vi "Manipulate_TDMS_files.vi"() -> ()   [LabVIEW 2015]
panel:
  in  "Group Name":bool
  in  "New Group Name":string
  out "Adding":bool
  out "Deleting":bool
  out "name2":string
  out "name 1":string
  in  "Add Button":bool
  in  "Open Button 2":bool
  in  "Listbox 2":i32[](listbox)=[9] caption="FreeRun_Beam_Tests_Int_Scint_2Apr2018.tdms"
  out "group names 2":string[](array[string])
  out "selected path 2":path caption="selected path"
  in  "Stop Button":bool
  in  "Remove Button":bool
  in  "Listbox":i32[](listbox)=[9] caption="FreeRun_Int_scint_new.tdms"
  in  "Open Button":bool
  out "group names":string[](array[string])
  out "selected path":path
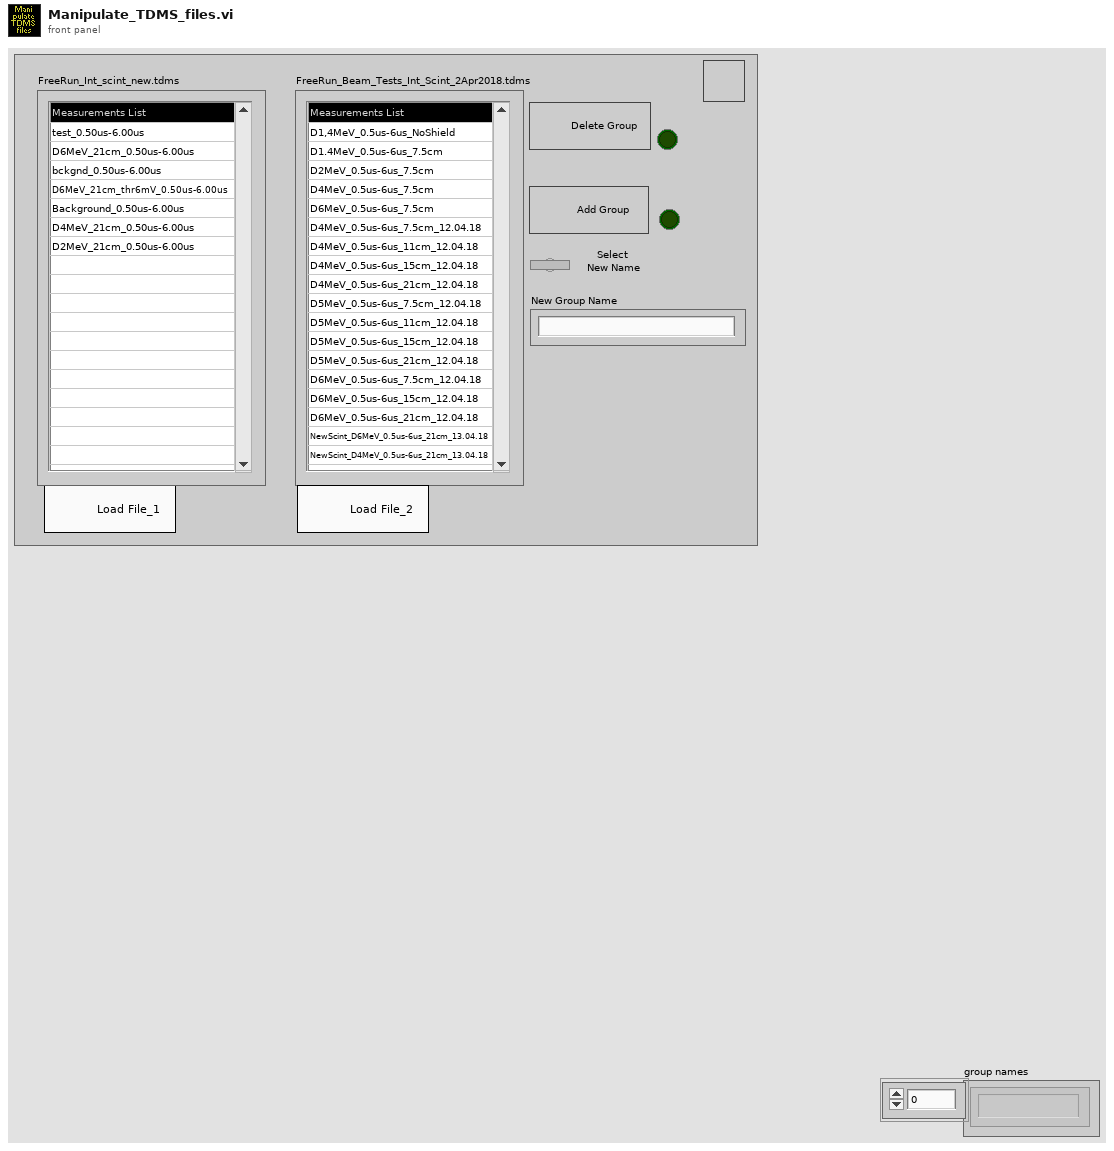
[diagram p1: front panel]
types:
  T1 = enum16{"open", "open or create", "create or replace", "create", "open (read-only)"}
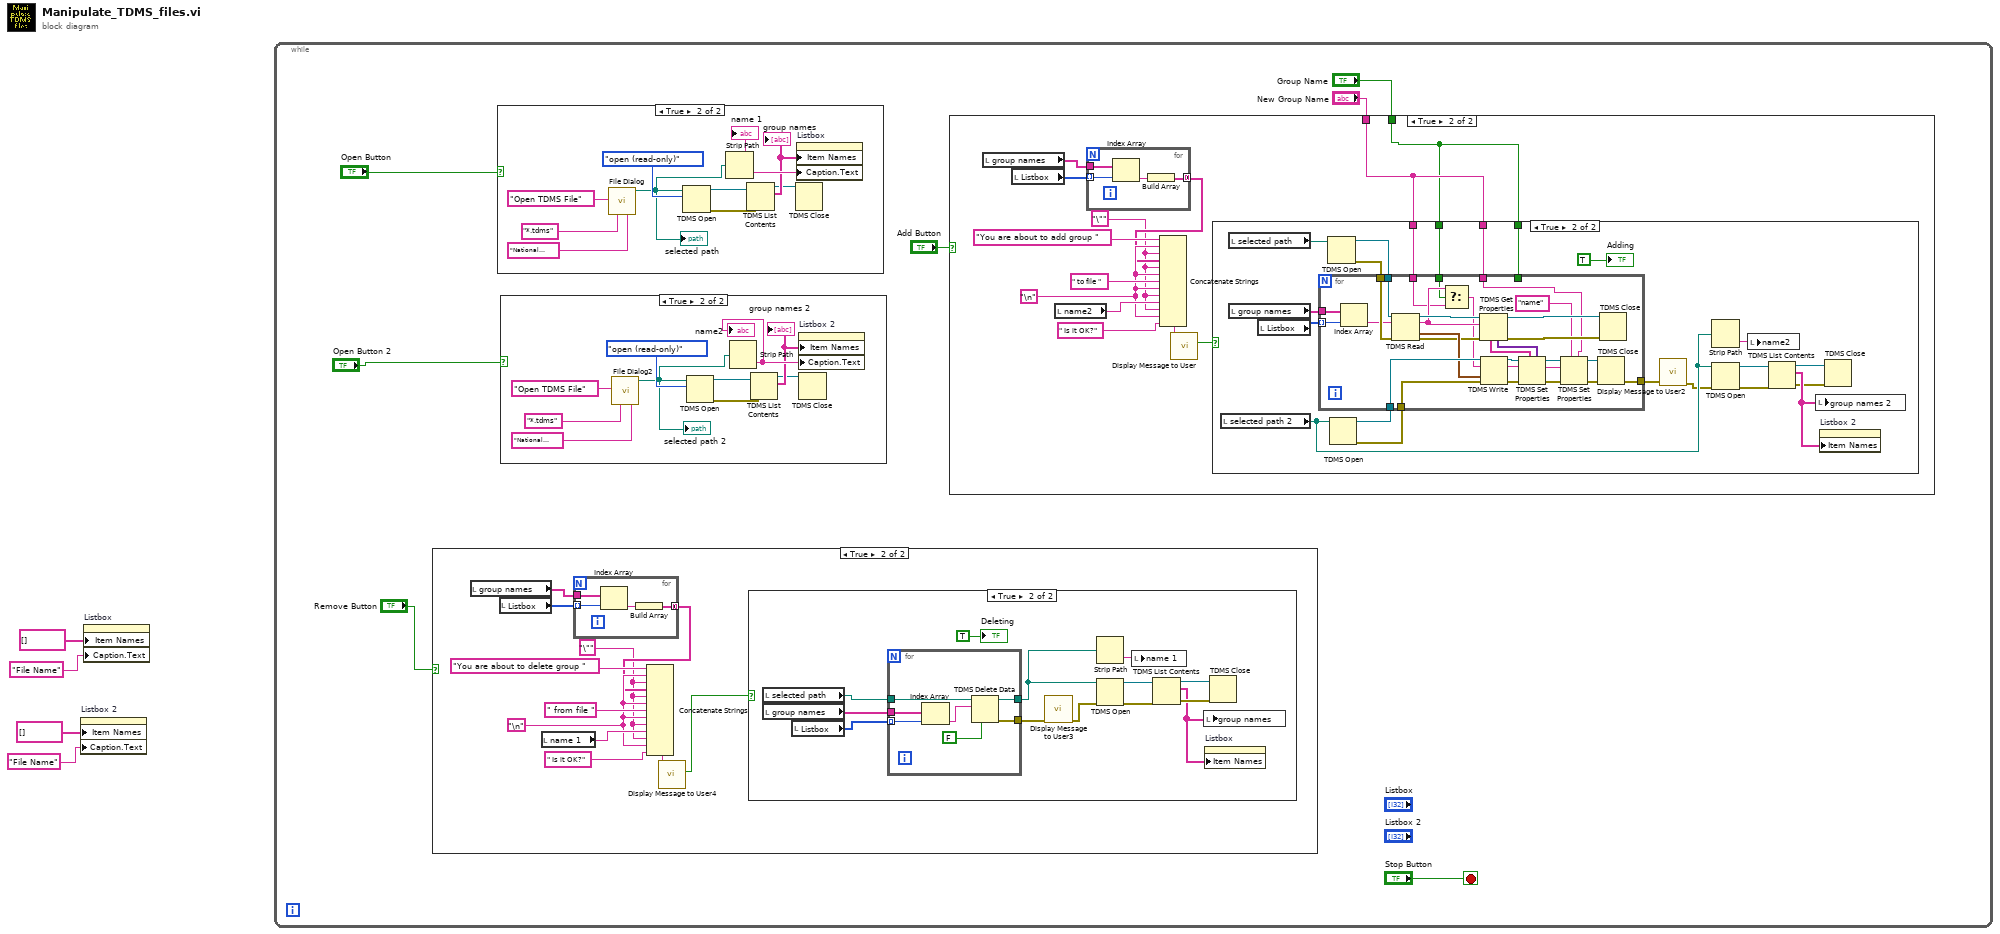
[diagram p0: block diagram]
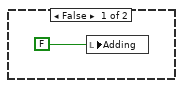
[diagram p2: hidden frame]
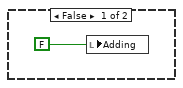
[diagram p3: hidden frame]
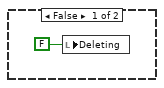
[diagram p5: hidden frame]
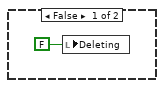
[diagram p6: hidden frame]
diagram:
  n1 = property on="Listbox 2" class="LstBox (strict)"("Item Names"=string[] [], "Caption.Text"="File Name") -> ()  [unwired: 2 in, 2 out]
  n2 = property on="Listbox" class="LstBox (strict)"("Item Names"=string[] [], "Caption.Text"="File Name") -> ()  [unwired: 2 in, 2 out]
  n3 = while {
    stop <- "Stop Button" stop-if-true
    n4 = case shown="True" "Remove Button" {
      frame False {
        n5 = local write "Deleting"(FALSE ("Deleting")) -> ()
      }
      frame True {
        w93 = "\""
        w95 = "\n"
        n6 = local read "group names"() -> (w101:string[])
        n7 = local read "Listbox"() -> (w100:i32[])
        n8 = local read "name 1"() -> (w99:string)
        n9 = for {
          tunnel: w101 -> [w106]
          tunnel: w100 -> [w105] mode=indexing
          tunnel: [w103] -> w94 mode=concatenating
          n10 = Index Array(array=w106, index=w105) -> (element=w104:string)
          n11 = Build Array(w104) -> (w103:string[])
        }
        n12 = Concatenate Strings("You are about to delete group " ("Message"), w95, w93, w94, w93, w95, " from file " ("Message"), w95, w93, w99, w93, w95, " Is it OK?" ("Message")) -> (w97:string)
        n13 = call "Display Message to User4"("Message"=w97) -> ("OK"=w92:bool)  [unwired: 9 in, 1 out]
        n14 = case shown="True" w92 {
          frame False {
            n15 = local write "Deleting"(FALSE ("Deleting")) -> ()
          }
          frame True {
            n16 = local read "selected path"() -> (w120:path)
            n17 = local read "group names"() -> (w119:string[])
            n18 = local read "Listbox"() -> (w118:i32[])
            n19 = for {
              tunnel: w120 -> [w127]
              tunnel: w119 -> [w126]
              tunnel: w118 -> [w125] mode=indexing
              tunnel: [w122] -> w117
              tunnel: [w121] -> w111
              n20 = Index Array(array=w126, index=w125) -> (element=w124:string)
              n21 = TDMS Delete Data(6:FALSE ("keep empty group/channel? (T)"), 10:w124, 11:w127) -> (0:w122:errorcluster, 3:w121:path)  [unwired: 4 in]
            }
            n22 = call "Display Message to User3"("error in (no error)"=w117) -> ("error out"=w108:errorcluster)  [unwired: 9 in, 1 out]
            n23 = Strip Path(path=w111) -> (name=w110:string)  [unwired: 1 out]
            n24 = TDMS Open(8:w108, 11:w111) -> (0:w114:errorcluster, 3:w115:refnum<k34>)  [unwired: 5 in]
            n25 = local write "name 1"(w110) -> ()
            n26 = TDMS List Contents(4:w114, 7:w115) -> (0:w112:errorcluster, 2:w109:string[], 3:w113:refnum<k34>)  [unwired: 1 in, 1 out]
            n27 = local write "group names"(w109) -> ()
            n28 = property on="Listbox" class="LstBox (strict)"("Item Names"=w109) -> ()  [unwired: 2 in, 2 out]
            n29 = TDMS Close(8:w112, 11:w113) -> ()  [unwired: 2 out]
            "Deleting" <- TRUE ("Deleting")
          }
        }
      }
    }
    n30 = case shown="True" "Open Button" {
      frame False {
      }
      frame True {
        n31 = call "File Dialog"("prompt"="Open TDMS File" ("prompt tdms"), "pattern (all files)"="*.tdms", "pattern label"="National Instruments TDM Streaming" ("pattern label tdms")) -> ("selected path"=w133:path)  [unwired: 4 in, 8 out]
        "selected path" <- w133
        n32 = TDMS Open(10:T1."open (read-only)" ("operation (0:open)"), 11:w133) -> (0:w129:errorcluster, 3:w130:refnum<k34>)  [unwired: 5 in]
        n33 = Strip Path(path=w133) -> (name=w132:string)  [unwired: 1 out]
        "name 1" <- w132
        n34 = TDMS List Contents(4:w129, 7:w130) -> (2:w131:string[], 3:w128:refnum<k34>)  [unwired: 1 in, 2 out]
        "group names" <- w131
        n35 = TDMS Close(11:w128) -> ()  [unwired: 1 in, 2 out]
        n36 = property on="Listbox" class="LstBox (strict)"("Item Names"=w131, "Caption.Text"=w132) -> ()  [unwired: 2 in, 2 out]
      }
    }
    n37 = case shown="True" "Open Button 2" {
      frame False {
      }
      frame True {
        n38 = call "File Dialog2"("prompt"="Open TDMS File" ("prompt tdms"), "pattern (all files)"="*.tdms", "pattern label"="National Instruments TDM Streaming" ("pattern label tdms")) -> ("selected path"=w86:path)  [unwired: 4 in, 8 out]
        "selected path 2" <- w86
        n39 = TDMS Open(10:T1."open (read-only)" ("operation (0:open)"), 11:w86) -> (0:w82:errorcluster, 3:w83:refnum<k34>)  [unwired: 5 in]
        n40 = Strip Path(path=w86) -> (name=w85:string)  [unwired: 1 out]
        "name2" <- w85
        n41 = TDMS List Contents(4:w82, 7:w83) -> (2:w84:string[], 3:w81:refnum<k34>)  [unwired: 1 in, 2 out]
        "group names 2" <- w84
        n42 = property on="Listbox 2" class="LstBox (strict)"("Item Names"=w84, "Caption.Text"=w85) -> ()  [unwired: 2 in, 2 out]
        n43 = TDMS Close(11:w81) -> ()  [unwired: 1 in, 2 out]
      }
    }
    n44 = case shown="True" "Add Button" {
      tunnel: "New Group Name" -> [_ w14]
      tunnel: "Group Name" -> [_ w13]
      frame False {
        n45 = local write "Adding"(FALSE ("Adding")) -> ()
      }
      frame True {
        w15 = "\""
        w17 = "\n"
        n46 = local read "group names"() -> (w23:string[])
        n47 = local read "Listbox"() -> (w22:i32[])
        n48 = local read "name2"() -> (w21:string)
        n49 = for {
          tunnel: w23 -> [w29]
          tunnel: w22 -> [w28] mode=indexing
          tunnel: [w26] -> w16 mode=concatenating
          n50 = Index Array(array=w29, index=w28) -> (element=w27:string)
          n51 = Build Array(w27) -> (w26:string[])
        }
        n52 = Concatenate Strings("You are about to add group " ("Message"), w17, w15, w16, w15, w17, " to file " ("Message"), w17, w15, w21, w15, w17, " Is it OK?" ("Message")) -> (w19:string)
        n53 = call "Display Message to User"("Message"=w19) -> ("OK"=w25:bool)  [unwired: 9 in, 1 out]
        n54 = case shown="True" w25 {
          tunnel: w14 -> [_ w34]
          tunnel: w14 -> [_ w33]
          tunnel: w13 -> [_ w32]
          tunnel: w13 -> [_ w31]
          frame False {
            n55 = local write "Adding"(FALSE ("Adding")) -> ()
          }
          frame True {
            n56 = local read "selected path 2"() -> (w36:path)
            n57 = local read "selected path"() -> (w51:path)
            n58 = local read "group names"() -> (w50:string[])
            n59 = local read "Listbox"() -> (w49:i32[])
            n60 = TDMS Open(11:w51) -> (0:w47:errorcluster, 3:w48:refnum<k34>)  [unwired: 6 in]
            n61 = TDMS Open(11:w36) -> (0:w45:errorcluster, 3:w46:refnum<k34>)  [unwired: 6 in]
            n62 = for {
              tunnel: w50 -> [w80]
              tunnel: w49 -> [w79] mode=indexing
              tunnel: w48 -> [w78]
              tunnel: w47 -> [w77]
              tunnel: w46 -> [w75]
              tunnel: w45 -> [w74]
              tunnel: [w72] -> w44
              tunnel: w34 -> [w52]
              tunnel: w33 -> [w62]
              tunnel: w32 -> [w61]
              tunnel: w31 -> [_]
              n63 = Index Array(array=w80, index=w79) -> (element=w76:string)
              n64 = TDMS Read(0:w78, 5:w76, 11:w77) -> (4:w71:refnum<k34>, 6:w63:string, 10:w73:waveform(dbl)[], 15:w69:errorcluster)  [unwired: 5 in, 2 out]
              n65 = Select(t=w63, s=w61, f=w62) -> (s? t:f=w54:string)
              n66 = TDMS Get Properties(8:w69, 10:w63, 11:w71) -> (0:w68:errorcluster, 3:w70:refnum<k34>, 4:w67:variant[], 6:w66:string[])  [unwired: 3 in, 2 out]
              n67 = TDMS Write(0:w75, 5:w54, 9:w73, 11:w74) -> (4:w65:refnum<k34>, 6:w60:string, 15:w64:errorcluster)  [unwired: 2 in, 1 out]
              n68 = TDMS Set Properties(5:w67, 7:w66, 8:w64, 10:w60, 11:w65) -> (0:w58:errorcluster, 2:w57:string, 3:w59:refnum<k34>)  [unwired: 1 in, 1 out]
              n69 = TDMS Set Properties(5:w52, 7:"name" ("channel name"), 8:w58, 10:w57, 11:w59) -> (0:w55:errorcluster, 3:w56:refnum<k34>)  [unwired: 1 in, 2 out]
              n70 = TDMS Close(8:w55, 11:w56) -> (0:w72:errorcluster)  [unwired: 1 out]
              n71 = TDMS Close(8:w68, 11:w70) -> ()  [unwired: 2 out]
            }
            n72 = call "Display Message to User2"("error in (no error)"=w44) -> ("error out"=w35:errorcluster)  [unwired: 9 in, 1 out]
            n73 = Strip Path(path=w36) -> (name=w41:string)  [unwired: 1 out]
            n74 = TDMS Open(8:w35, 11:w36) -> (0:w38:errorcluster, 3:w37:refnum<k34>)  [unwired: 5 in]
            n75 = local write "name2"(w41) -> ()
            n76 = TDMS List Contents(4:w38, 7:w37) -> (0:w40:errorcluster, 2:w42:string[], 3:w39:refnum<k34>)  [unwired: 1 in, 1 out]
            n77 = local write "group names 2"(w42) -> ()
            n78 = property on="Listbox 2" class="LstBox (strict)"("Item Names"=w42) -> ()  [unwired: 2 in, 2 out]
            n79 = TDMS Close(8:w40, 11:w39) -> ()  [unwired: 2 out]
            "Adding" <- TRUE ("Adding")
          }
        }
      }
    }
  }
